vi "Proportional Cal.vi"(10 "PID gains":T1, 11 "Error":dbl) -> (3 "Proportional Term":dbl)   [LabVIEW 2023]
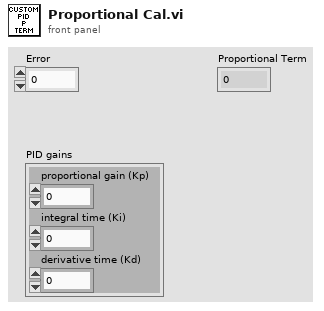
[diagram p1: front panel]
types:
  T1 = cluster{"proportional gain (Kp)":dbl, "integral time (Ki)":dbl, "derivative time (Kd)":dbl}
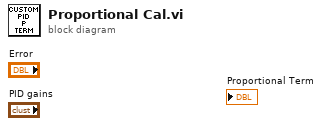
[diagram p0: block diagram]
diagram:
